vi "Set_Source_Exported_Assembly_VI_Data.vi"(8 "error in (no error)":errorcluster, 10 "ExportAssemblyVIinfo":T1, 11 "AB_Source_Exported_Assembly_VI.lvclass in":refnum<class "AB_Source_Exported_Assembly_VI.lvclass">) -> (0 "error out":errorcluster, 3 "AB_Source_Exported_Assembly_VI.lvclass out":refnum<class "AB_Source_Exported_Assembly_VI.lvclass">)   [LabVIEW 2020, in "AB_Source_Exported_Assembly_VI.lvclass"]
uses:
  <vilib>/AppBuilder/AB_Classes/Source/ExportedAssemblyVI/AB_Source_Exported_Assembly_VI.lvclass
  <vilib>/AppBuilder/AB_InteropAssembly_DistVI_Proto_Info.ctl
  <vilib>/AppBuilder/IOStatus.ctl
  <vilib>/AppBuilder/AB_Classes/Source/ExportedAssemblyVI/AB_Source_Exported_Assembly_VI.lvclass/AB_Source_Exported_Assembly_VI.ctl
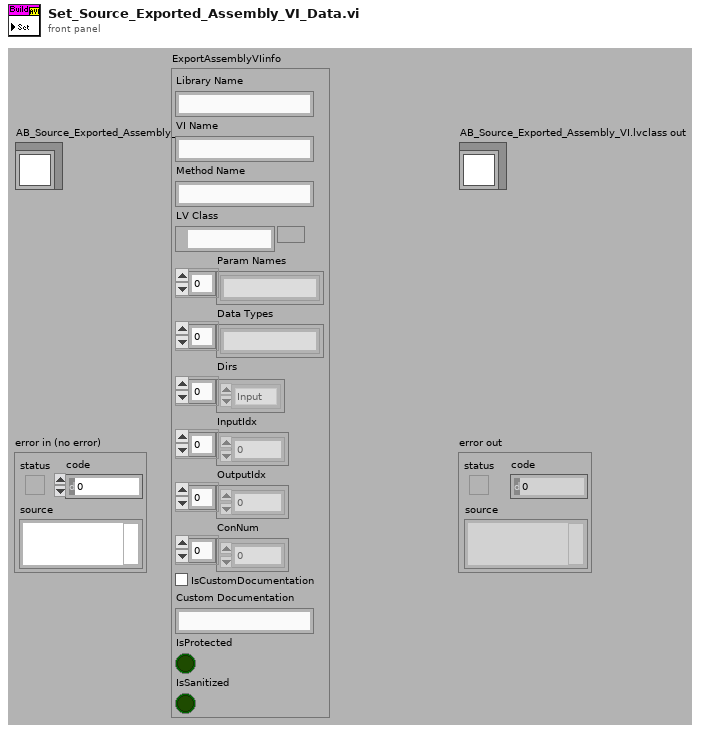
[diagram p1: front panel]
types:
  T1 = typedef "AB_InteropAssembly_DistVI_Proto_Info.ctl" = cluster{"Library Name":string, "VI Name":string, "Method Name":string, "LV Class":path, "Param Names":string[], "Data Types":string[], "Dirs":T2[], "InputIdx":i32[], "OutputIdx":i32[], "ConNum":i8[], "IsCustomDocumentation":bool, "Custom Documentation":string, "IsProtected":bool, "IsSanitized":bool}
  T2 = typedef "IOStatus.ctl" = enum16{"Input", "Output", "Input/Output", "InputDeleted", "OutputDeleted", "IODeleted", "ErrorClusterIn", "ErrorClusterOut"}
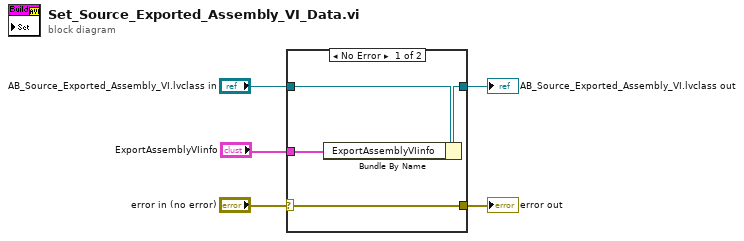
[diagram p0: block diagram]
diagram:
  n1 = case shown="No Error" "error in (no error)" {
    selector: "error in (no error)" -> [w9 w10]
    tunnel: [w9 w10] -> w4
    tunnel: [w7 w11] -> w2
    tunnel: "AB_Source_Exported_Assembly_VI.lvclass in" -> [w8 w11]
    tunnel: "ExportAssemblyVIinfo" -> [w6 _]
    frame No Error {
      n2 = Bundle By Name(cluster=w8, "ExportAssemblyVIinfo"=w6) -> (w7:refnum<class "AB_Source_Exported_Assembly_VI.lvclass">)
    }
    frame Error {
    }
  }
  "error out" <- w4
  "AB_Source_Exported_Assembly_VI.lvclass out" <- w2
